vi "init.vi"(8 "error in (no error)":errorcluster, 9 "activeMQ_dll_directory":path, 10 "brokerConnectionString":string) -> (0 "error out":errorcluster, 2 "messageEvent":refnum<user-event>, 3 "ActiveMQBroker out":refnum<class "ActiveMQBroker.lvclass">)   [LabVIEW 2024, in "ActiveMQBroker.lvclass"]
uses:
  ActiveMQBroker.lvclass
  ActiveMQBroker.lvclass/ActiveMQBroker.ctl
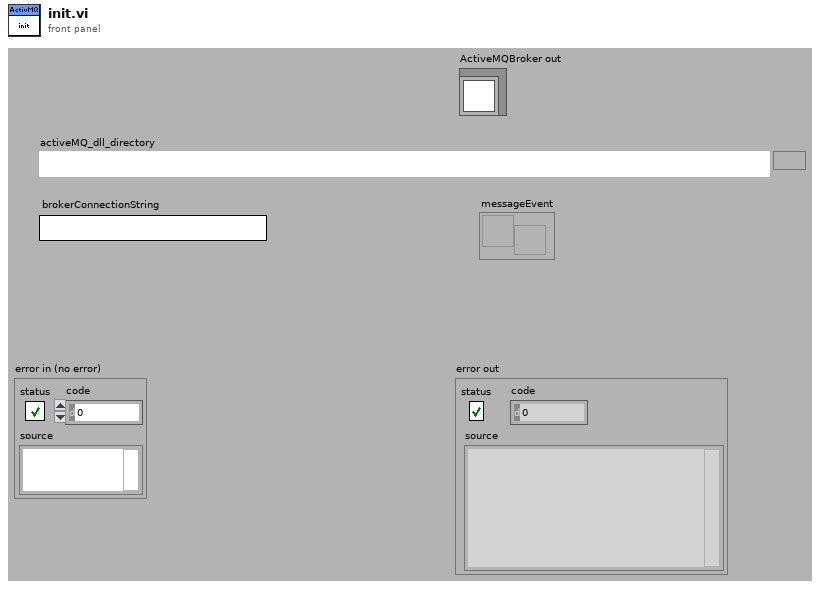
[diagram p1: front panel]
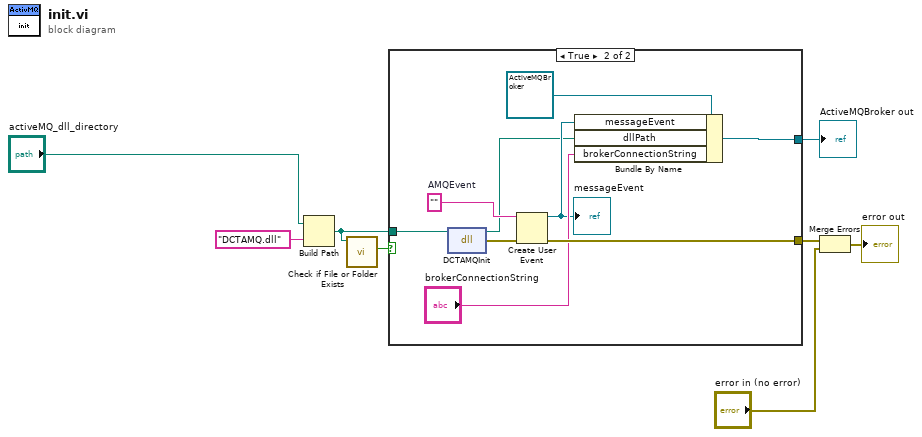
[diagram p0: block diagram]
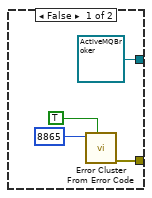
[diagram p2: hidden frame]
diagram:
  n1 = Build Path(base path="activeMQ_dll_directory", name or relative path="DCTAMQ.dll") -> (appended path=w3:path)
  n2 = call <vilib>:"Check if File or Folder Exists.vi"("path"=w3) -> ("file or folder exists?"=w2:bool)  [unwired: 8 in, 2 out]
  n3 = case shown="True" w2 {
    tunnel: [refnum<class "ActiveMQBroker.lvclass"> refnum ("ActiveMQBroker in") w20] -> w8
    tunnel: [w10 w19] -> w5
    tunnel: w3 -> [_ w15]
    frame False {
      n4 = call <vilib>:"Error Cluster From Error Code.vi"("show call chain? (False)"=TRUE, "error code (0)"=8865) -> ("error out"=w10:errorcluster)  [unwired: 7 in]
    }
    frame True {
      w21 = ""  # AMQEvent
      n5 = dll-call lib="?" fn="DCTAMQInit"(path in=w15) -> (path out=w13:path, error out=w14:errorcluster)  [unwired: 3 in]
      n6 = Create User Event(user event datatype=w21, error in=w14) -> (user event=w17:refnum<user-event>, error out=w19:errorcluster)
      "messageEvent" <- w17
      n7 = Bundle By Name(cluster=refnum<class "ActiveMQBroker.lvclass"> refnum ("ActiveMQBroker in"), "messageEvent"=w17, "dllPath"=w13, "brokerConnectionString"="brokerConnectionString") -> (w20:refnum<class "ActiveMQBroker.lvclass">)
    }
  }
  "ActiveMQBroker out" <- w8
  n8 = Merge Errors(w5, "error in (no error)") -> (→"error out":errorcluster)
